vi "DM_Control_AE.vi"(0 "Mirror ID":string, 1 "Action":enum16{"WRITE", "READ"}(ring), 11 "Mirror Control IN":T1 {"Modes"."Amplititude" step=0.05}) -> (4 "Mirror ID Out":string, 15 "Mirror Control OUT":T1 {"Modes"."Amplititude" step=0.05})   [LabVIEW 2014]
uses:
  DMControl_V3.ctl
panel:
  in  "Mirror Data Holder":cluster{"Top Mirror":T1, "Bottom Mirror":T1} {"Bottom Mirror"."Modes"."Amplititude" step=0.05; "Top Mirror"."Modes"."Amplititude" step=0.05}
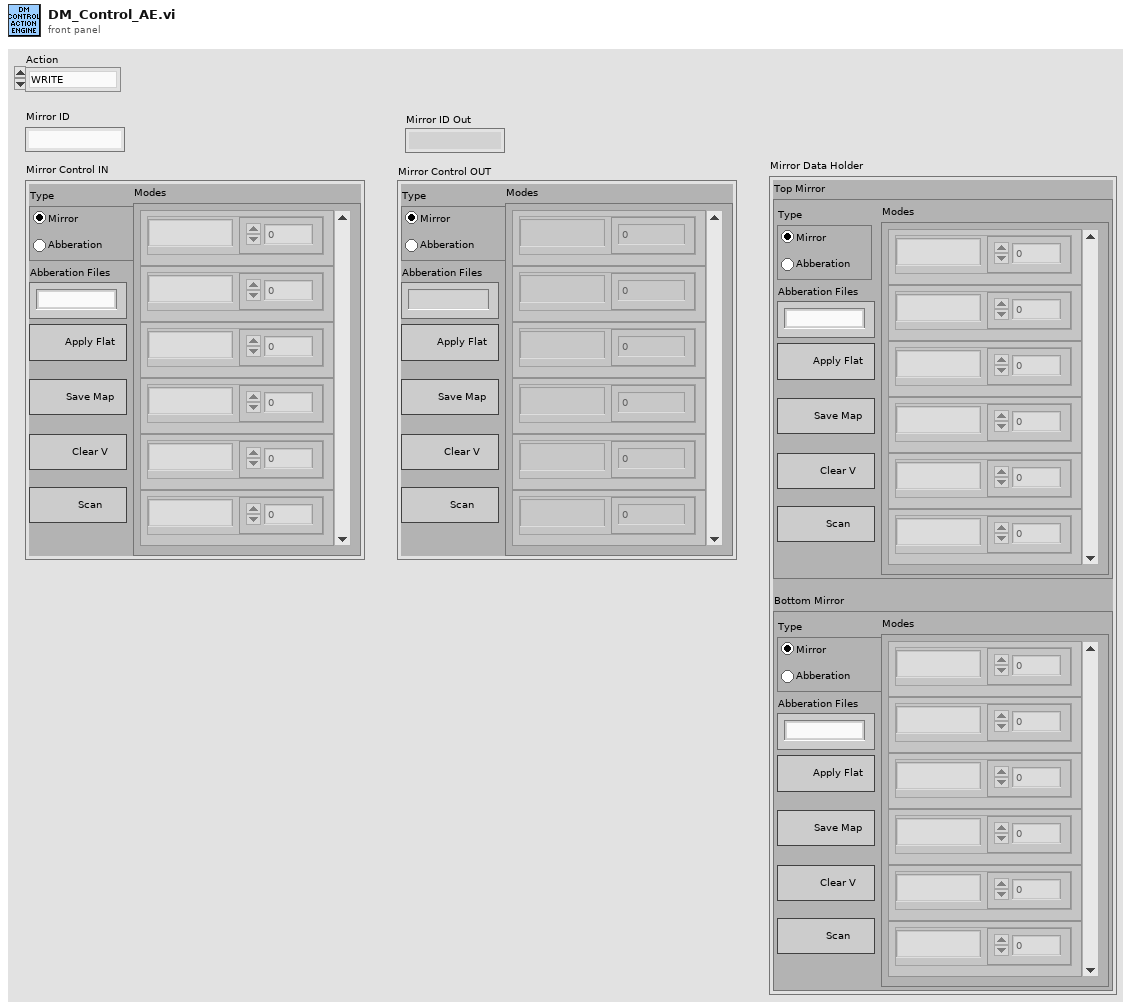
[diagram p1: front panel]
types:
  T1 = typedef "DMControl_V3.ctl" = cluster{"Type":enum32{"Mirror", "Abberation"}, "Modes":cluster{"Mode":string, "Amplititude":dbl}[], "Apply Flat":bool, "Save Map":bool, "Clear Voltage":bool, "Abberation Files":u16, "Scan ":bool}
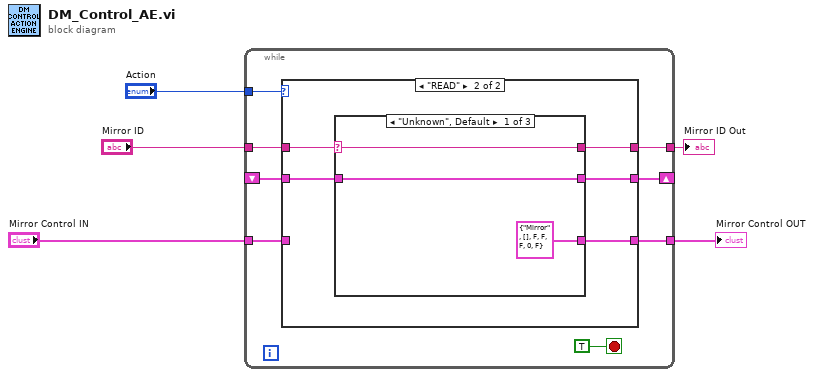
[diagram p0: block diagram]
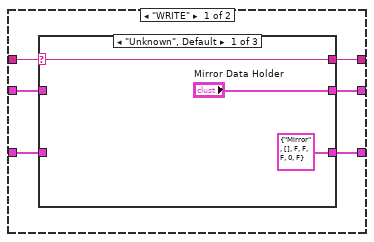
[diagram p2: hidden frame]
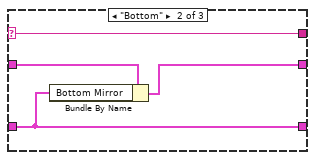
[diagram p3: hidden frame]
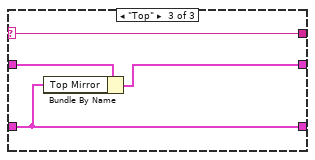
[diagram p4: hidden frame]
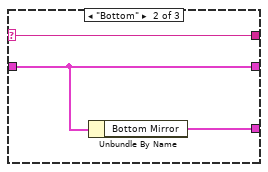
[diagram p5: hidden frame]
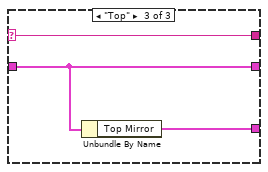
[diagram p6: hidden frame]
diagram:
  n1 = while {
    tunnel: "Action" -> [w12]
    tunnel: "Mirror Control IN" -> [w11]
    tunnel: "Mirror ID" -> [w10]
    tunnel: [w9] -> w1
    tunnel: [w8] -> w2
    shift-right: [w7] -> _
    shift-left: _ -> [w6]
    stop <- TRUE stop-if-true
    n2 = case shown="\"READ\"" w12 {
      tunnel: w11 -> [w18 _]
      tunnel: w10 -> [w19 w35]
      tunnel: [w17 w34] -> w9
      tunnel: [w16 w33] -> w8
      tunnel: [w15 w31] -> w7
      tunnel: w6 -> [w14 w32]
      frame "WRITE" {
        n3 = case shown="\"Unknown\", Default" w19 {
          selector: w19 -> [w21 w26 w30]
          tunnel: w18 -> [_ w25 w29]
          tunnel: [T1 {"Type"=enum."Mirror", "Modes"=[], "Apply Flat"=FALSE, "Save Map"=FALSE, "Clear Voltage"=FALSE, "Abberation Files"=0, "Scan "=FALSE} ("Control") w25 w29] -> w17
          tunnel: [w21 w26 w30] -> w16
          tunnel: ["Mirror Data Holder" w23 w28] -> w15
          tunnel: w14 -> [_ w24 w27]
          frame "Unknown", Default {
          }
          frame "Bottom" {
            n4 = Bundle By Name(cluster=w24, "Bottom Mirror"=w25) -> (w23:cluster{"Top Mirror":T1, "Bottom Mirror":T1})
          }
          frame "Top" {
            n5 = Bundle By Name(cluster=w27, "Top Mirror"=w29) -> (w28:cluster{"Top Mirror":T1, "Bottom Mirror":T1})
          }
        }
      }
      frame "READ" {
        n6 = case shown="\"Unknown\", Default" w35 {
          selector: w35 -> [w36 w39 w42]
          tunnel: [w38 w41 w44] -> w31
          tunnel: w32 -> [w38 w41 w44]
          tunnel: [T1 {"Type"=enum."Mirror", "Modes"=[], "Apply Flat"=FALSE, "Save Map"=FALSE, "Clear Voltage"=FALSE, "Abberation Files"=0, "Scan "=FALSE} ("Top") w40 w43] -> w34
          tunnel: [w36 w39 w42] -> w33
          frame "Unknown", Default {
          }
          frame "Bottom" {
            n7 = Unbundle By Name(w41) -> ("Bottom Mirror"=w40:T1)
          }
          frame "Top" {
            n8 = Unbundle By Name(w44) -> ("Top Mirror"=w43:T1)
          }
        }
      }
    }
  }
  "Mirror ID Out" <- w2
  "Mirror Control OUT" <- w1
